vi "Read Exposure Time.vi"(8 "error in (no error)":errorcluster, 10 "Shutter-NP In":T1, 11 "Container in":refnum<class "Container.lvclass">) -> (0 "error out":errorcluster, 2 "Shutter-NP Out":T1, 3 "Container out":refnum<class "Container.lvclass">)   [LabVIEW 2016, in "Container.lvclass"]
uses:
  Container.lvclass
  Controls/Shutters.ctl
  Controls/Shutter Data.ctl
  Controls/Shutter States.ctl
  Container.lvclass/Container.ctl
  ExtFlat/ExtFlatShutt.lvclass
  LFCSim/LFCSimShutt.lvclass
  Sci/SciShutt.lvclass
  SimFlat/SimFlatShutt.lvclass
  Solar/CalShutt.lvclass
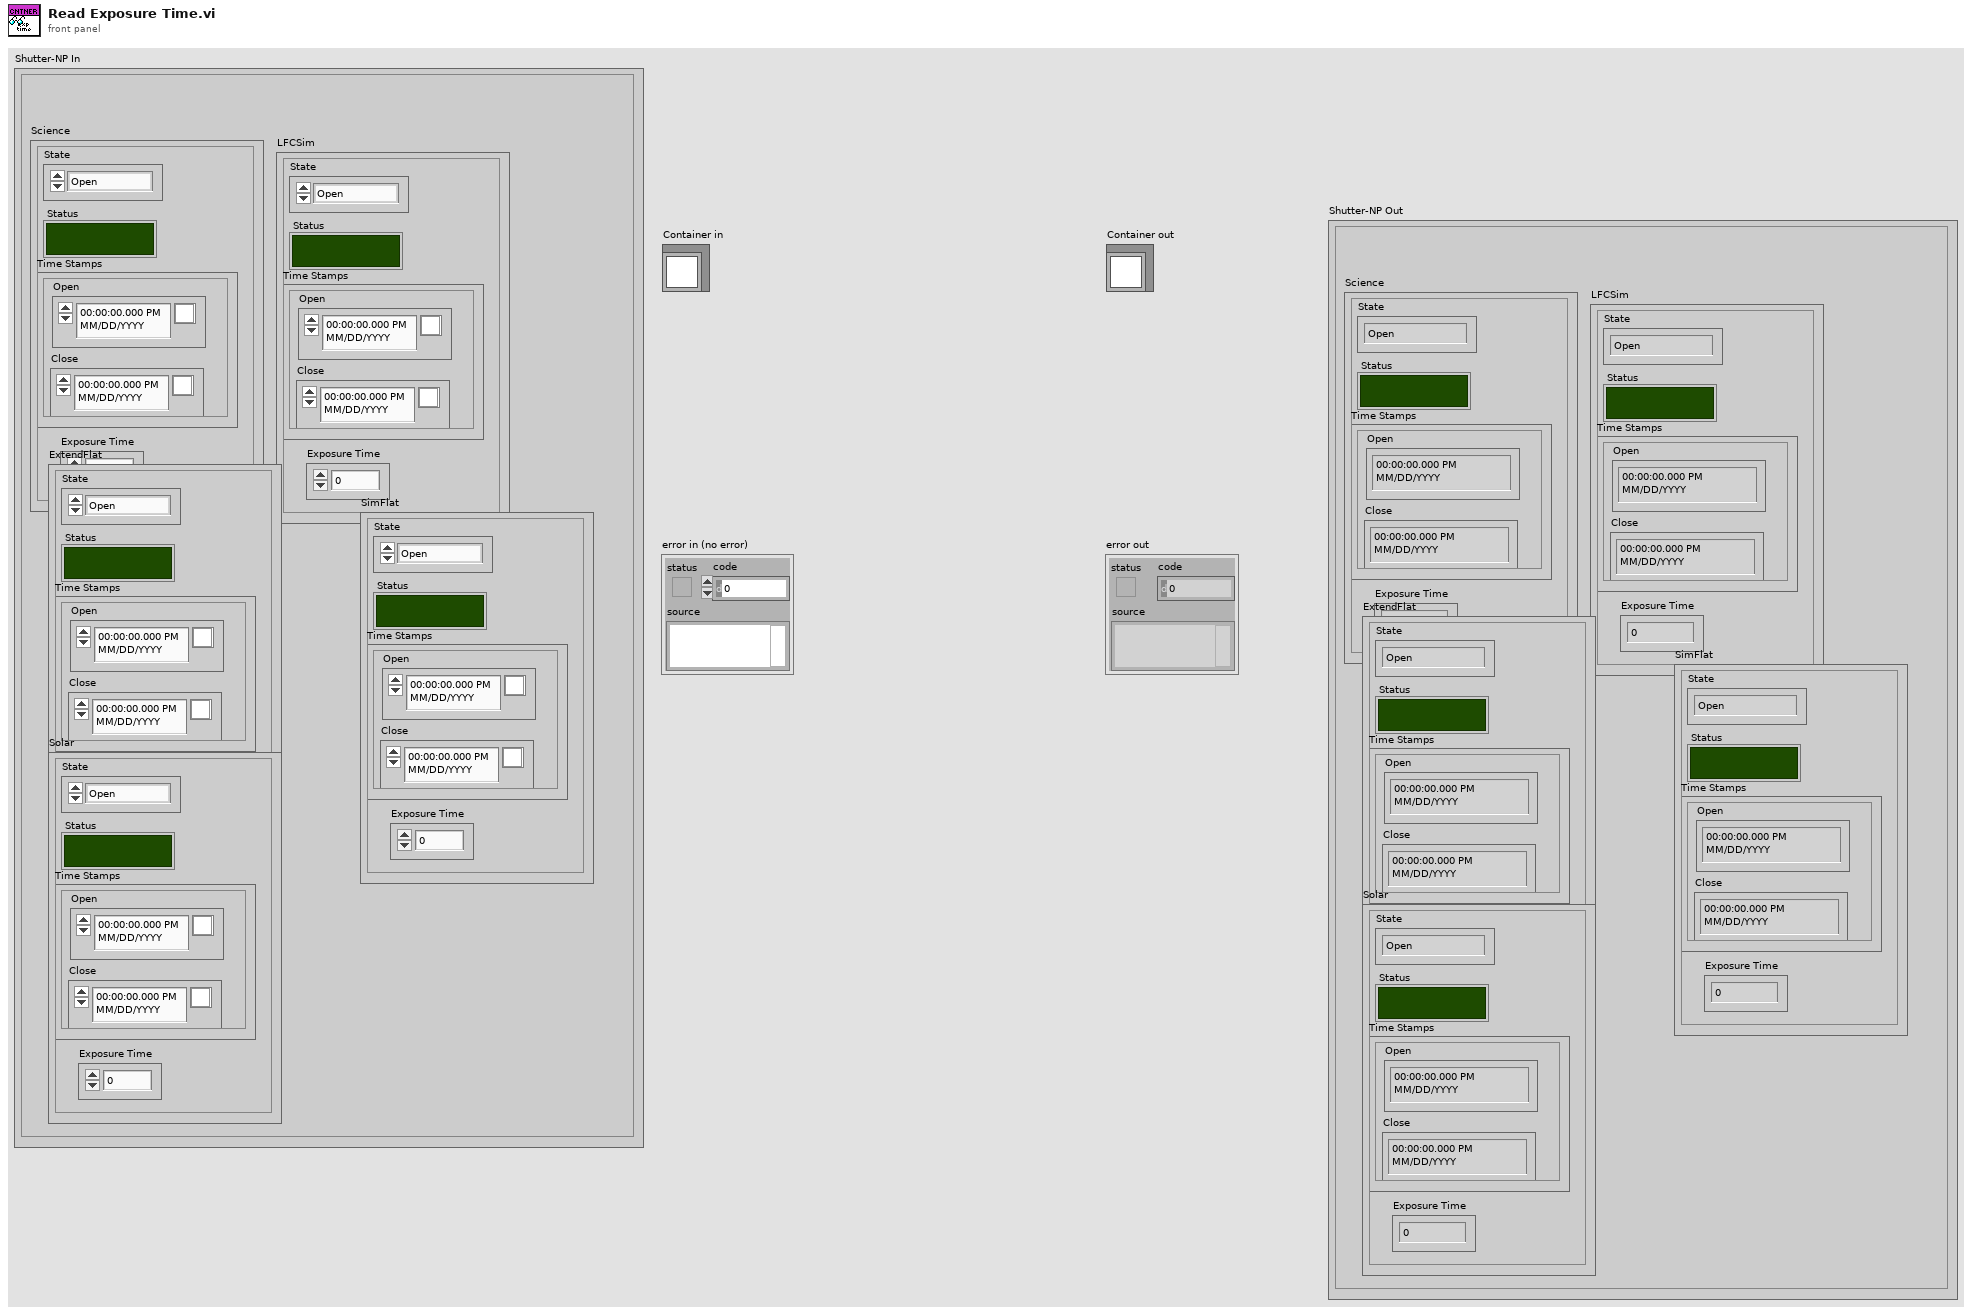
[diagram p1: front panel]
types:
  T1 = typedef "Shutters.ctl" = cluster{"Science":T2, "LFCSim":T2, "ExtendFlat":T2, "SimFlat":T2, "Solar":T2}
  T2 = typedef "Shutter Data.ctl" = cluster{"Status":bool, "State":T3, "Time Stamps":cluster{"Open":timestamp, "Close":timestamp}, "Exposure Time":dbl}
  T3 = typedef "Shutter States.ctl" = enum16{"Open", "Close", "Wait", "Off", "Arm", "Idle"}
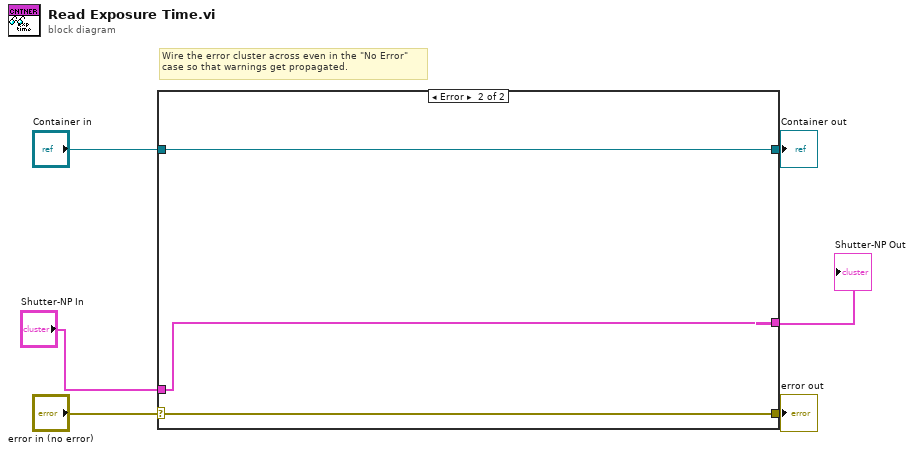
[diagram p0: block diagram]
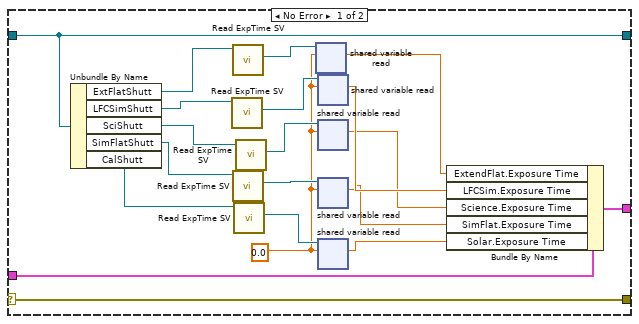
[diagram p2: hidden frame]
diagram:
  # "Wire the error cluster across even in the \"No Error\"\ncase so that warnings get propagated."
  n1 = case shown="Error" "error in (no error)" {
    selector: "error in (no error)" -> [w26 w29]
    tunnel: [w26 w29] -> w5
    tunnel: [w25 w28] -> w3
    tunnel: "Container in" -> [w25 w28]
    tunnel: "Shutter-NP In" -> [w13 w27]
    tunnel: [w7 w27] -> w1
    frame No Error {
      w14 = 0.0
      n2 = Unbundle By Name(w25) -> ("ExtFlatShutt"=w24:refnum<class "ExtFlatShutt.lvclass">, "LFCSimShutt"=w23:refnum<class "LFCSimShutt.lvclass">, "SciShutt"=w22:refnum<class "SciShutt.lvclass">, "SimFlatShutt"=w21:refnum<class "SimFlatShutt.lvclass">, "CalShutt"=w20:refnum<class "CalShutt.lvclass">)
      n3 = call-dynamic "Read ExpTime SV.vi"("Integrator in"=w23) -> ("ExpTime SV"=w16:refnum<k21>)  [unwired: 8 in, 2 out]
      n4 = call-dynamic "Read ExpTime SV.vi"("Integrator in"=w24) -> ("ExpTime SV"=w19:refnum<k21>)  [unwired: 8 in, 2 out]
      n5 = call-dynamic "Read ExpTime SV.vi"("Integrator in"=w21) -> ("ExpTime SV"=w15:refnum<k21>)  [unwired: 8 in, 2 out]
      n6 = call-dynamic "Read ExpTime SV.vi"("Integrator in"=w20) -> ("ExpTime SV"=w18:refnum<k21>)  [unwired: 8 in, 2 out]
      n7 = call-dynamic "Read ExpTime SV.vi"("Integrator in"=w22) -> ("ExpTime SV"=w17:refnum<k21>)  [unwired: 8 in, 2 out]
      n8 = shared-variable-read(w19, w14) -> (w12:dbl)  [unwired: 1 in, 3 out]
      n9 = shared-variable-read(w16, w14) -> (w11:dbl)  [unwired: 1 in, 3 out]
      n10 = shared-variable-read(w17, w14) -> (w10:dbl)  [unwired: 1 in, 3 out]
      n11 = shared-variable-read(w15, w14) -> (w9:dbl)  [unwired: 1 in, 3 out]
      n12 = shared-variable-read(w18, w14) -> (w8:dbl)  [unwired: 1 in, 3 out]
      n13 = Bundle By Name(cluster=w13, "ExtendFlat.Exposure Time"=w12, "LFCSim.Exposure Time"=w11, "Science.Exposure Time"=w10, "SimFlat.Exposure Time"=w9, "Solar.Exposure Time"=w8) -> (w7:T1)
    }
    frame Error {
    }
  }
  "error out" <- w5
  "Container out" <- w3
  "Shutter-NP Out" <- w1
